vi "Teleop.vi"(10 "Match Info":T1={"Autonomous Elapsed Seconds"=0.0, "TeleOp Elapsed Seconds"=0.0, "Disabled Elapsed Seconds"=0.0, "Visited Autonomous"=FALSE, "Visited TeleOp"=FALSE, "Visited Disabled"=FALSE, "Autonomous Settings"={"Autonomous Style"=enum."Independent", "VI Refnum"=refnum}}, 11 "Call Context":T2) -> ()   [LabVIEW 2019]
doc: "This VI is called for each enabled TeleOp packet received from the DS. It is typically used to read from joysticks and other inputs and update I/O or setpoints for timed control loops. It should complete and return within 20 milliseconds or risk missing DS packets."
uses:
  <vilib>/Rock Robotics/WPI/DriverStation/WPI_DriverStationDerivedRobotMode.ctl
  <vilib>/Rock Robotics/WPI/DriverStation/WPI_DriverStationMatch Info.ctl
  <vilib>/Rock Robotics/WPI/Utilities/WPI_GetSetVariantRefNum.vi
  <vilib>/Rock Robotics/Network Tables/NT Write Boolean Array.vi
  <vilib>/Rock Robotics/Network Tables/NT Write Numeric Array.vi
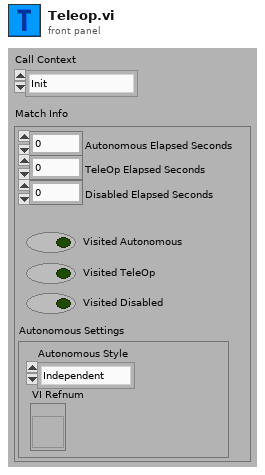
[diagram p1: front panel]
types:
  T1 = typedef "WPI_DriverStationMatch Info.ctl" = cluster{"Autonomous Elapsed Seconds":dbl, "TeleOp Elapsed Seconds":dbl, "Disabled Elapsed Seconds":dbl, "Visited Autonomous":bool, "Visited TeleOp":bool, "Visited Disabled":bool, "Autonomous Settings":cluster{"Autonomous Style":enum16{"Iterative", "Independent"}, "VI Refnum":refnum<vi>}}
  T2 = typedef "WPI_DriverStationDerivedRobotMode.ctl" = enum16{"Init", "Execute", "Stop"}
  T3 = typedef "WPI_JoystickDevRef.ctl" = cluster{"Device":T4}
  T4 = typedef "WPI_JoystickDeviceEnum.ctl" = enum16{"USB 0", "USB 1", "USB 2", "USB 3", "USB 4", "USB 5"}
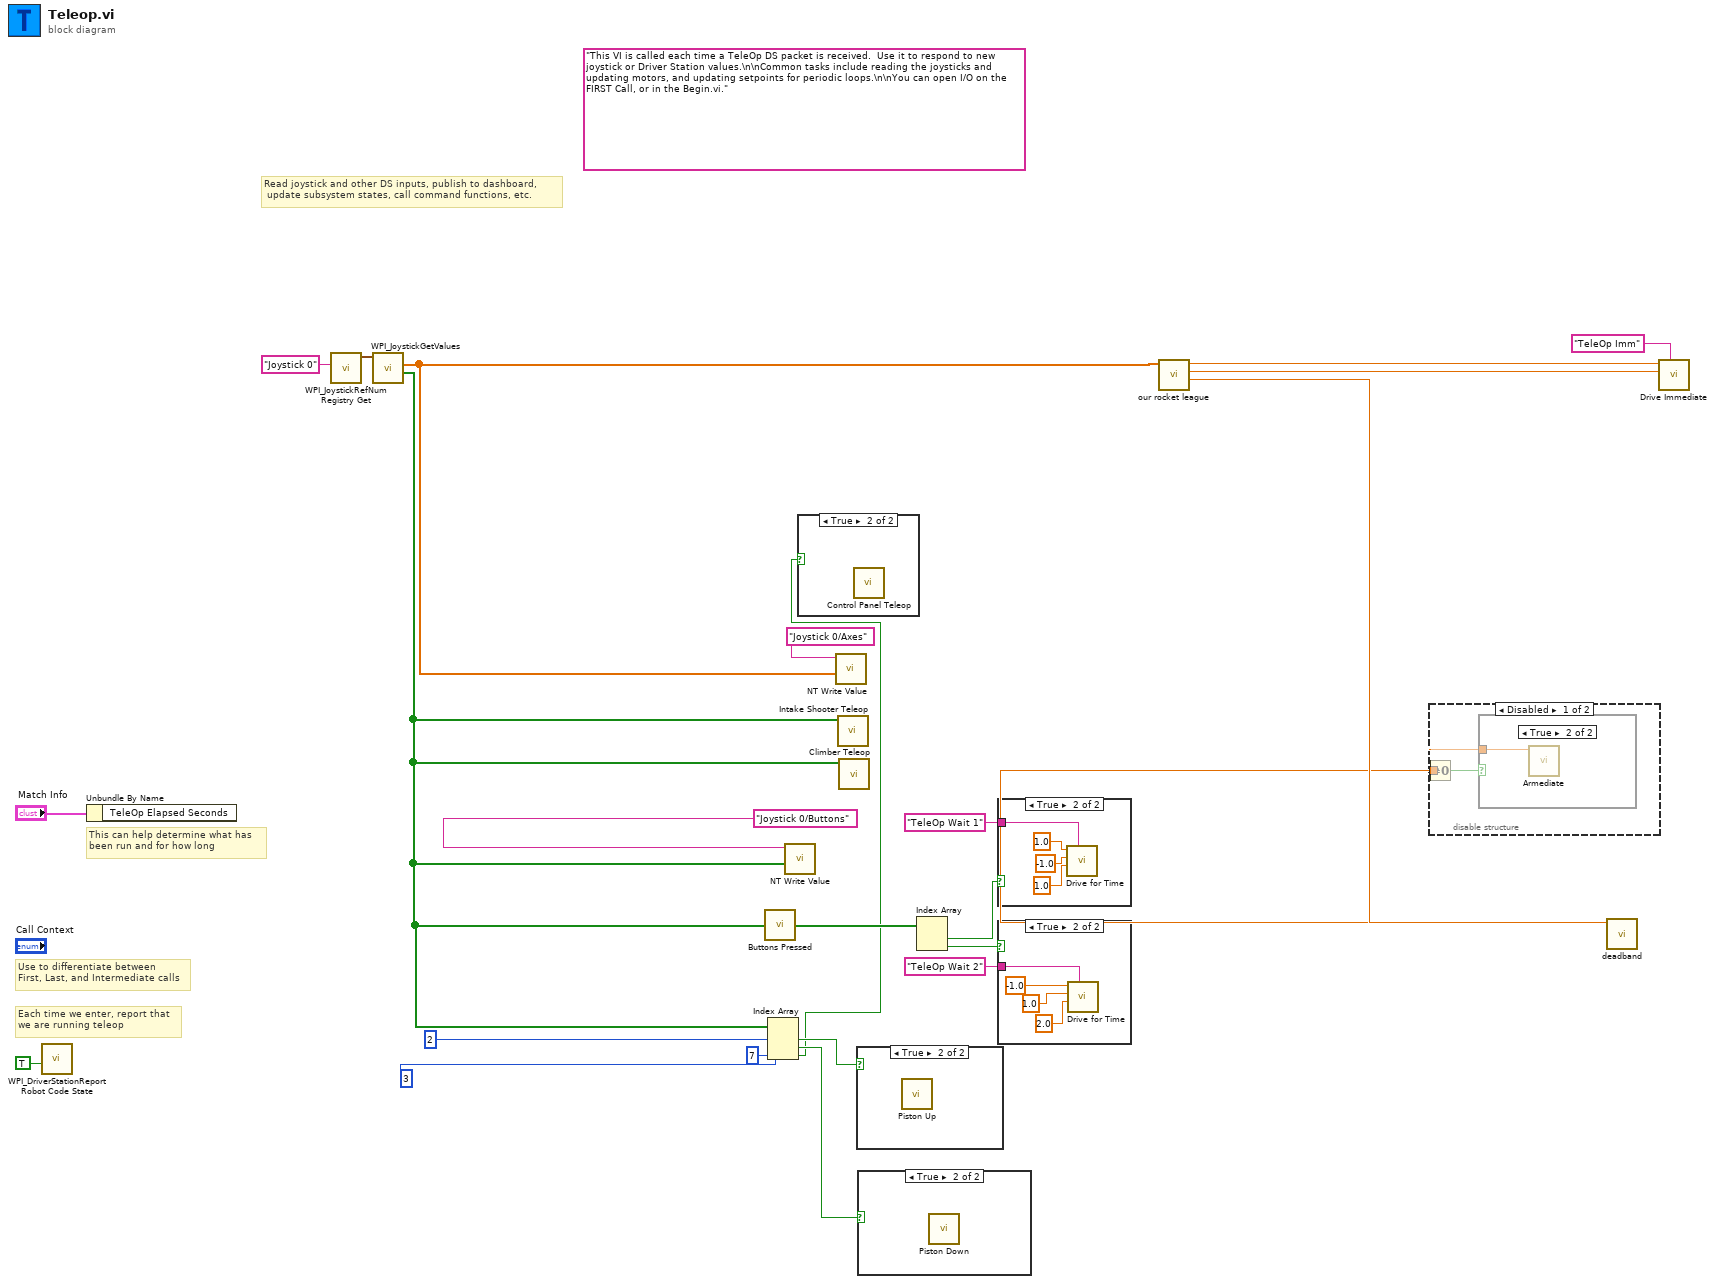
[diagram p0: block diagram]
diagram:
  (unwired) "This VI is called each time a TeleOp DS packet is received.  Use it to respond to new joystick or Driver Station values.\n\nCommon tasks include reading the joysticks and updating motors, and updating setpoints for periodic loops.\n\nYou can open I/O on the FIRST Call, or in the Begin.vi."
  # "Read joystick and other DS inputs, publish to dashboard,\n update subsystem states, call command functions, etc."
  # "Each time we enter, report that\nwe are running teleop"
  # "Use to differentiate between\nFirst, Last, and Intermediate calls"
  # "This can help determine what has\nbeen run and for how long"
  n1 = call <vilib>:"WPI_DriverStationReport Robot Code State.vi"("TeleOp"=TRUE ("Autonomous")) -> ()  [unwired: 10 in, 1 out]
  n2 = Unbundle By Name("Match Info") -> ()  [unwired: 1 out]
  n3 = call <vilib>:"WPI_JoystickRefNum Registry Get.vi"("refnum name"="Joystick 0") -> ("JoystickDevRef"=w21:T3)  [unwired: 1 in, 9 out]
  n4 = call <vilib>:"WPI_JoystickGetValues.vi"("JoystickDevRef"=w21) -> ("Buttons"=w10:bool[], "Axes"=w14:dbl[])  [unwired: 6 in, 3 out]
  n5 = call "Buttons Pressed.vi"("Button Values"=w10) -> ("Button Presses"=w13:bool[])
  n6 = Index Array(array=w10, index #1=2 ("index"), index #2=3 ("index"), index #3=7 ("index")) -> (element #1=w7:bool, element #2=w6:bool, element #3=w1:bool)
  n7 = call-poly <vilib>:"NT Write Value.vi"("Boolean Array"=w10, "Name"="Joystick 0/Buttons") -> ()  [unwired: 9 in, 1 out]
  n8 = case shown="True" w1 {
    frame False {
    }
    frame True {
      n9 = call "Control Panel Teleop.vi"() -> ()  [unwired: 12 in]
    }
  }
  n10 = call-poly <vilib>:"NT Write Value.vi"("Numeric Array"=w14, "Name"="Joystick 0/Axes") -> ()  [unwired: 9 in, 1 out]
  n11 = call "Intake Shooter Teleop.vi"("Buttons"=w10) -> ()  [unwired: 11 in]
  n12 = call "Climber Teleop.vi"("Buttons"=w10) -> ()  [unwired: 11 in]
  n13 = case shown="True" w7 {
    frame False {
    }
    frame True {
      n14 = call "Piston Up.vi"() -> ()  [unwired: 11 in, 1 out]
    }
  }
  n15 = case shown="True" w6 {
    frame False {
    }
    frame True {
      n16 = call "Piston Down.vi"() -> ()  [unwired: 11 in, 1 out]
    }
  }
  n17 = Index Array(array=w13) -> (element #1=w18:bool, element #2=w17:bool)  [unwired: 2 in]
  n18 = case shown="True" w18 {
    tunnel: "TeleOp Wait 1" ("Description") -> [_ w27]
    frame False {
    }
    frame True {
      n19 = call "Drive for Time.vi"("Description"=w27, "Seconds"=1.0, "Right Speed"=-1.0, "Left Speed"=1.0) -> ()  [unwired: 7 in, 1 out]
    }
  }
  n20 = case shown="True" w17 {
    tunnel: "TeleOp Wait 2" ("Description") -> [_ w30]
    frame False {
    }
    frame True {
      n21 = call "Drive for Time.vi"("Description"=w30, "Seconds"=2.0, "Right Speed"=1.0, "Left Speed"=-1.0) -> ()  [unwired: 7 in, 1 out]
    }
  }
  n22 = call "our rocket league.vi"("Axes"=w14) -> ("upper limit"=w12:dbl, "upper limit 2"=w3:dbl, "upper limit 3"=w4:dbl)  [unwired: 8 in]
  n23 = call "deadband.vi"("Joystick Value"=w12) -> ("Val"=w11:dbl)  [unwired: 10 in]
  n24 = disable-structure shown="Disabled" {
    disable-tunnel: w11 -> [w33 _]
    frame Disabled {
      n25 = Not Equal To 0?(x=w33) -> (x != 0?=w34:bool)
      n26 = case shown="True" w34 {
        tunnel: w33 -> [_ w35]
        frame False {
        }
        frame True {
          n27 = call "Armediate.vi"("Setpoint"=w35) -> ()  [unwired: 10 in, 1 out]
        }
      }
    }
    frame Enabled {
    }
  }
  n28 = call "Drive Immediate.vi"("Description"="TeleOp Imm", "Right Setpoint"=w3, "Left Setpoint"=w4) -> ()  [unwired: 8 in, 1 out]
